vi "Leader.vi"   [LabVIEW 2016]
uses:
  <vilib>/NXT/Block Support/NXT_TimerIndex.ctl
  <vilib>/NXT/Block Support/NXT_OutputPort.ctl
  <vilib>/NXT/Subs/MotorOutput.ctl
  <vilib>/NXT/Dual Mode Library/Sensors/Reset_Timer.vi
  <vilib>/NXT/Dual Mode Library/Sensors/Read_Timer.vi
  <vilib>/NXT/Dual Mode Library/Motors/ResetMotor.vi
  <vilib>/NXT/Dual Mode Library/Motors/Rotation.vi
  <vilib>/NXT/NXTIO Xnodes/NXTIONodeSubVIs/NXTMoveMotors.vi
  <vilib>/NXT/Dual Mode Library/Display/drawNumber_float.vi
  <vilib>/NXT/NXTIO Xnodes/NXTIONodeSubVIs/NXTStopMotors.vi
  <vilib>/NXT/Dual Mode Library/Display/drawText.vi
  <vilib>/NXT/Dual Mode Library/Display/drawNumber.vi
  <vilib>/NXT/Dual Mode Library/Display/drawText_Right.vi
  <vilib>/NXT/Subs/LVHSConnector.ctl
  <vilib>/NXT/NXTIO Xnodes/AddressXNode/NXTIOAddress.xnode
  <vilib>/NXT/NXTIO Xnodes/NXTIOXNode/NXTIO.xnode
  <vilib>/NXT/LegoClasses/BrickReference/BrickReference.lvclass
types:
  T1 = typedef "NXT_TimerIndex.ctl" = u8
  T2 = typedef "LVHSConnector.ctl" = refnum<class "BrickReference.lvclass">
  T3 = typedef "NXT_OutputPort.ctl" = u8
  T4 = typedef "MotorOutput.ctl" = u8
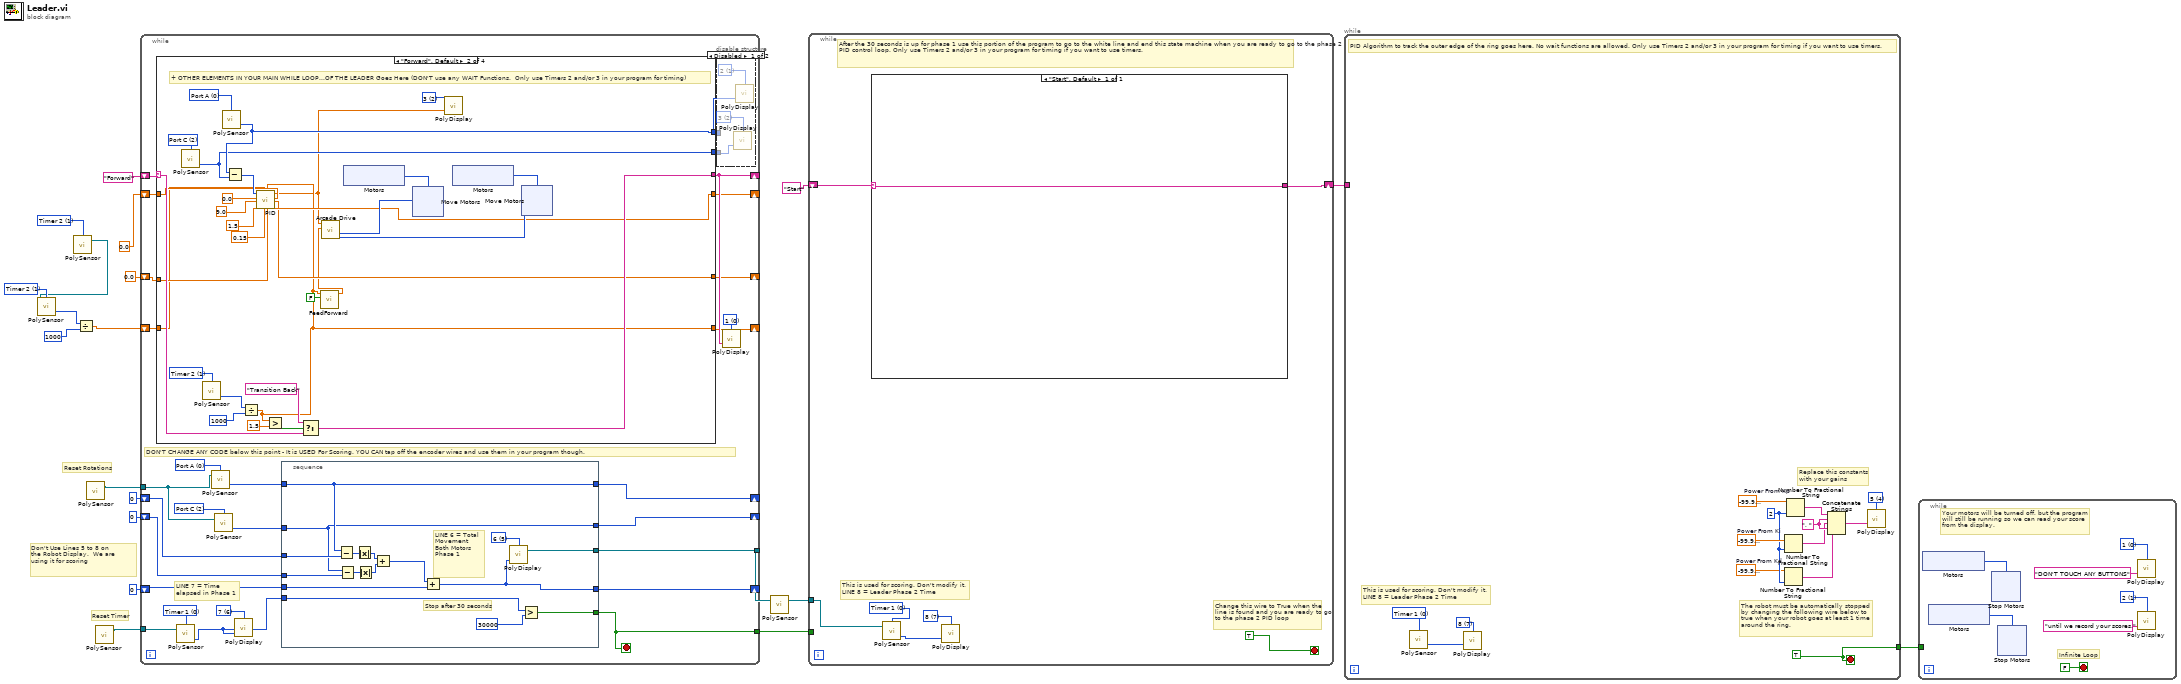
[diagram p0: block diagram]
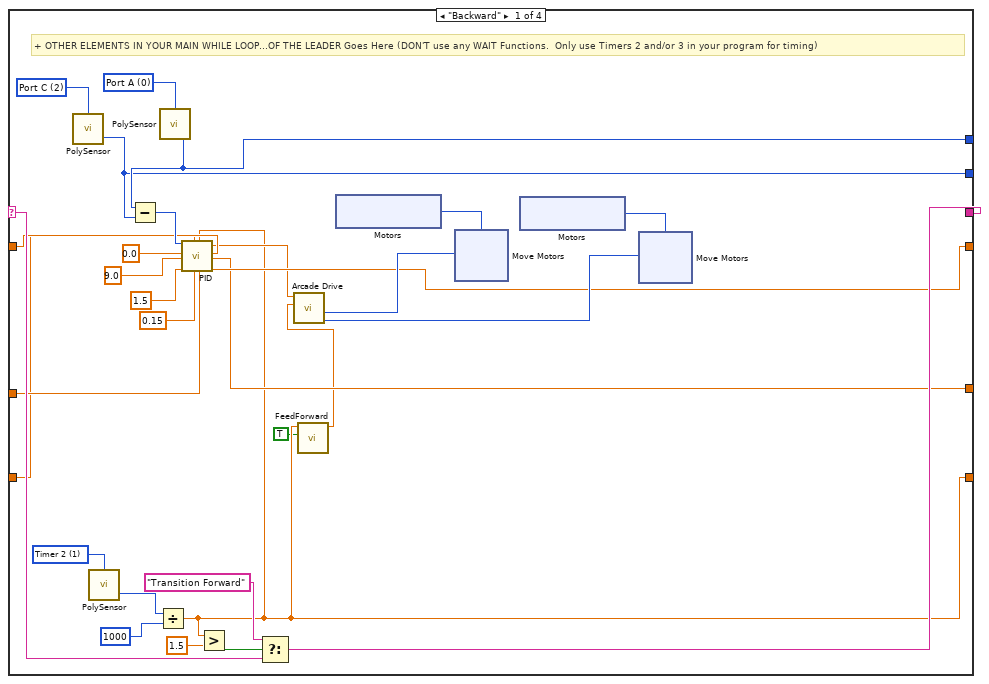
[diagram p3: hidden frame]
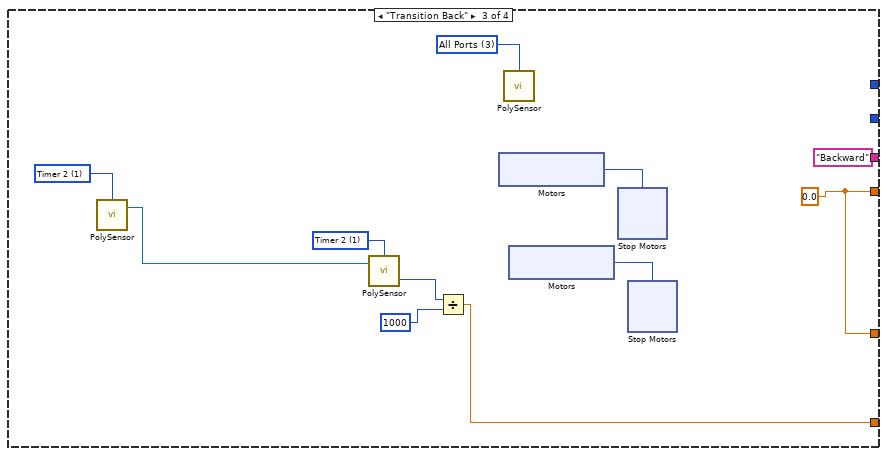
[diagram p4: hidden frame]
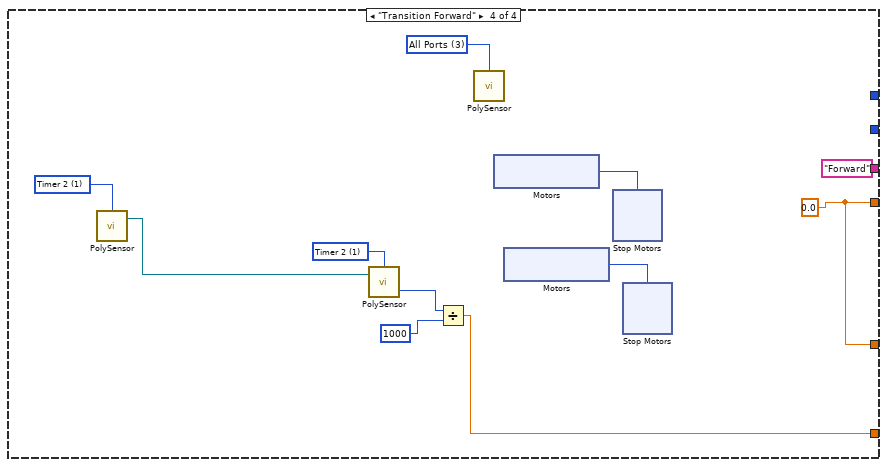
[diagram p5: hidden frame]
diagram:
  w4 = T1 1 items=["Timer 1", "Timer 2", "Timer 3"] ("Timer (Timer 1)")
  w8 = T1 1 items=["Timer 1", "Timer 2", "Timer 3"] ("Timer (Timer 1)")
  # "Don't Use Lines 5 to 8 on\nthe Robot Display.  We are \nusing it for scoring"
  # "Reset Timer"
  # "Reset Rotations"
  n1 = call-poly <vilib>:"PolySensor.vi"("Timer (Timer 1)"=w8) -> ("NXT/EV3"=w2:T2)  [unwired: 3 in]
  n2 = call-poly <vilib>:"PolySensor.vi"("NXT/EV3"=w2, "Timer (Timer 1)"=w4) -> ("Value (msec)"=w5:u32)  [unwired: 1 in, 1 out]
  n3 = Divide(x=w5, y=u32 1000) -> (x/y=w1:dbl)
  n4 = call-poly <vilib>:"PolySensor.vi"() -> ("NXT/EV3"=w16:T2)  [unwired: 4 in]
  n5 = call-poly <vilib>:"PolySensor.vi"() -> ("NXT/EV3"=w15:T2)  [unwired: 4 in]
  n6 = while {
    tunnel: w16 -> [w48]
    shift-right: [w40] -> _
    shift-left: 0 ("Angle of Rotation") -> [w42]
    shift-right: [w39] -> _
    shift-left: 0 ("Angle of Rotation") -> [w41]
    shift-right: [w46] -> _
    shift-left: 0 -> [w47]
    tunnel: w15 -> [w36]
    tunnel: [w45] -> w13
    shift-right: [w29] -> _
    shift-left: "Forward" -> [w38]
    tunnel: [w31] -> w12
    shift-right: [w27] -> _
    shift-left: 0.0 ("Accumulate In") -> [w28]
    shift-right: [w25] -> _
    shift-left: 0.0 ("Accumulate In") -> [w26]
    shift-right: [w23] -> _
    shift-left: w1 -> [w24]
    stop <- w45 stop-if-true
    w30 = i16 0 items=["1", "2", "3", "4", "5", "6", "7", "8", "9", "10", "11", "12"] ("Line")
    w33 = i16 6 items=["1", "2", "3", "4", "5", "6", "7", "8", "9", "10", "11", "12"] ("Line")
    w34 = T3 0 items=["Port A", "Port B", "Port C", "Port D"] ("Port (Port A)")
    w35 = T3 2 items=["Port A", "Port B", "Port C", "Port D"] ("Port (Port A)")
    w37 = T1 0 items=["Timer 1", "Timer 2", "Timer 3"] ("Timer (Timer 1)")
    # "DON'T CHANGE ANY CODE below this point - It is USED For Scoring. YOU CAN tap off the encoder wires and use them in your program though."
    # "LINE 7 = Time elapsed in Phase 1"
    n7 = case shown="\"Forward\", Default" w38 {
      selector: w38 -> [w77 w124 _ _]
      tunnel: [w78 w125 "Backward" ("t") "Forward" ("t")] -> w29
      tunnel: w28 -> [w63 w110 _ _]
      tunnel: [w61 w108 w154 w177] -> w27
      tunnel: w26 -> [w60 w107 _ _]
      tunnel: [w62 w109 w154 w177] -> w25
      tunnel: w24 -> [w59 w106 _ _]
      tunnel: [w55 w103 w149 w172] -> w23
      tunnel: [w58 w105 _ _] -> w22
      tunnel: [w57 w104 _ _] -> w21
      frame "Backward" {
        w72 = T3 2 items=["Port A", "Port B", "Port C", "Port D"] ("Port (Port A)")
        w73 = T3 0 items=["Port A", "Port B", "Port C", "Port D"] ("Port (Port A)")
        w80 = T1 1 items=["Timer 1", "Timer 2", "Timer 3"] ("Timer (Timer 1)")
        # "+ OTHER ELEMENTS IN YOUR MAIN WHILE LOOP...OF THE LEADER Goes Here (DON'T use any WAIT Functions.  Only use Timers 2 and/or 3 in your program for timing)"
        n8 = call-poly <vilib>:"PolySensor.vi"("Port (Port A)"=w72) -> ("Angle of Rotation"=w57:i32)  [unwired: 2 in, 1 out]
        n9 = call-poly <vilib>:"PolySensor.vi"("Timer (Timer 1)"=w80) -> ("Value (msec)"=w71:u32)  [unwired: 2 in, 1 out]
        n10 = Divide(x=w71, y=u32 1000) -> (x/y=w55:dbl)
        n11 = call-poly <vilib>:"PolySensor.vi"("Port (Port A)"=w73) -> ("Angle of Rotation"=w58:i32)  [unwired: 2 in, 1 out]
        n12 = Subtract(x=w58, y=w57) -> (x-y=w68:i32)
        n13 = call "PID.vi"("Sensor Input"=w68, "Setpoint"=0.0, "Kp"=9.0, "Ki"=1.5, "Prev Time"=w59, "Kd"=0.15, "Curr Time"=w55, "Accumulate In"=w63, "Previous Error"=w60) -> ("Output Val"=w56:dbl, "Accumulate Out"=w61:dbl, "Current Error"=w62:dbl)  [unwired: 5 in, 3 out]
        n14 = Greater?(x=w55, y=1.5) -> (0:w79:bool)
        n15 = Select(t="Transition Forward", s=w79, f=w77) -> (s? t:f=w78:string)
        n16 = call "FeedForward.vi"("backward?"=TRUE, "Current Time"=w55) -> ("f(t)"=w54:sgl)  [unwired: 9 in]
        n17 = call "Arcade Drive.vi"("Drive"=w54, "Rotate"=w56) -> ("Left Motor"=w74:i8, "Right Motor"=w75:i8)  [unwired: 8 in]
        n18 = xnode "Motors"() -> ("Motor"=w81:T3)
        n19 = xnode "Move Motors"("Power/Speed 1"=w75, "Motors"=w81) -> ()  [unwired: 1 in, 1 out]
        n20 = xnode "Motors"() -> ("Motor"=w82:T3)
        n21 = xnode "Move Motors"("Power/Speed 1"=w74, "Motors"=w82) -> ()  [unwired: 1 in, 1 out]
      }
      frame "Forward", Default {
        w99 = i16 2 items=["1", "2", "3", "4", "5", "6", "7", "8", "9", "10", "11", "12"] ("Line")
        w119 = T3 2 items=["Port A", "Port B", "Port C", "Port D"] ("Port (Port A)")
        w120 = T3 0 items=["Port A", "Port B", "Port C", "Port D"] ("Port (Port A)")
        w127 = T1 1 items=["Timer 1", "Timer 2", "Timer 3"] ("Timer (Timer 1)")
        # "+ OTHER ELEMENTS IN YOUR MAIN WHILE LOOP...OF THE LEADER Goes Here (DON'T use any WAIT Functions.  Only use Timers 2 and/or 3 in your program for timing)"
        n22 = call-poly <vilib>:"PolySensor.vi"("Port (Port A)"=w119) -> ("Angle of Rotation"=w104:i32)  [unwired: 2 in, 1 out]
        n23 = call-poly <vilib>:"PolySensor.vi"("Timer (Timer 1)"=w127) -> ("Value (msec)"=w118:u32)  [unwired: 2 in, 1 out]
        n24 = call-poly <vilib>:"PolySensor.vi"("Port (Port A)"=w120) -> ("Angle of Rotation"=w105:i32)  [unwired: 2 in, 1 out]
        n25 = Subtract(x=w105, y=w104) -> (x-y=w115:i32)
        n26 = Divide(x=w118, y=u32 1000) -> (x/y=w103:dbl)
        n27 = call "PID.vi"("Sensor Input"=w115, "Setpoint"=0.0, "Kp"=9.0, "Ki"=1.5, "Prev Time"=w106, "Kd"=0.15, "Curr Time"=w103, "Accumulate In"=w110, "Previous Error"=w107) -> ("Output Val"=w100:dbl, "Accumulate Out"=w108:dbl, "Current Error"=w109:dbl)  [unwired: 5 in, 3 out]
        n28 = Greater?(x=w103, y=1.5) -> (0:w126:bool)
        n29 = Select(t="Transition Back", s=w126, f=w124) -> (s? t:f=w125:string)
        n30 = call "FeedForward.vi"("backward?"=FALSE, "Current Time"=w103) -> ("f(t)"=w101:sgl)  [unwired: 9 in]
        n31 = call "Arcade Drive.vi"("Drive"=w101, "Rotate"=w100) -> ("Left Motor"=w121:i8, "Right Motor"=w122:i8)  [unwired: 8 in]
        n32 = xnode "Motors"() -> ("Motor"=w128:T3)
        n33 = xnode "Move Motors"("Power/Speed 1"=w122, "Motors"=w128) -> ()  [unwired: 1 in, 1 out]
        n34 = call-poly <vilib>:"PolyDisplay.vi"("number"=w100, "Line"=w99) -> ()  [unwired: 2 in, 1 out]
        n35 = xnode "Motors"() -> ("Motor"=w129:T3)
        n36 = xnode "Move Motors"("Power/Speed 1"=w121, "Motors"=w129) -> ()  [unwired: 1 in, 1 out]
      }
      frame "Transition Back" {
        w148 = T4 3 items=["Port A"=0, "Port B"=1, "Port C"=2, "Ports A & B"=4, "Ports A & C"=5, "Ports B & C"=6, "All Ports"=3] ("Port (All Ports)")
        w152 = T1 1 items=["Timer 1", "Timer 2", "Timer 3"] ("Timer (Timer 1)")
        w154 = 0.0 ("Accumulate In")
        w156 = T1 1 items=["Timer 1", "Timer 2", "Timer 3"] ("Timer (Timer 1)")
        n37 = call-poly <vilib>:"PolySensor.vi"("Timer (Timer 1)"=w156) -> ("NXT/EV3"=w150:T2)  [unwired: 3 in]
        n38 = call-poly <vilib>:"PolySensor.vi"("NXT/EV3"=w150, "Timer (Timer 1)"=w152) -> ("Value (msec)"=w151:u32)  [unwired: 1 in, 1 out]
        n39 = Divide(x=w151, y=u32 1000) -> (x/y=w149:dbl)
        n40 = xnode "Motors"() -> ("Motor"=w147:T3)
        n41 = call-poly <vilib>:"PolySensor.vi"("Port (All Ports)"=w148) -> ()  [unwired: 3 in, 1 out]
        n42 = xnode "Motors"() -> ("Motor"=w146:T3)
        n43 = xnode "Stop Motors"("Motors"=w147) -> ()  [unwired: 1 in, 1 out]
        n44 = xnode "Stop Motors"("Motors"=w146) -> ()  [unwired: 1 in, 1 out]
      }
      frame "Transition Forward" {
        w171 = T4 3 items=["Port A"=0, "Port B"=1, "Port C"=2, "Ports A & B"=4, "Ports A & C"=5, "Ports B & C"=6, "All Ports"=3] ("Port (All Ports)")
        w175 = T1 1 items=["Timer 1", "Timer 2", "Timer 3"] ("Timer (Timer 1)")
        w177 = 0.0 ("Accumulate In")
        w179 = T1 1 items=["Timer 1", "Timer 2", "Timer 3"] ("Timer (Timer 1)")
        n45 = call-poly <vilib>:"PolySensor.vi"("Timer (Timer 1)"=w179) -> ("NXT/EV3"=w173:T2)  [unwired: 3 in]
        n46 = call-poly <vilib>:"PolySensor.vi"("NXT/EV3"=w173, "Timer (Timer 1)"=w175) -> ("Value (msec)"=w174:u32)  [unwired: 1 in, 1 out]
        n47 = Divide(x=w174, y=u32 1000) -> (x/y=w172:dbl)
        n48 = call-poly <vilib>:"PolySensor.vi"("Port (All Ports)"=w171) -> ()  [unwired: 3 in, 1 out]
        n49 = xnode "Motors"() -> ("Motor"=w170:T3)
        n50 = xnode "Motors"() -> ("Motor"=w169:T3)
        n51 = xnode "Stop Motors"("Motors"=w170) -> ()  [unwired: 1 in, 1 out]
        n52 = xnode "Stop Motors"("Motors"=w169) -> ()  [unwired: 1 in, 1 out]
      }
    }
    n53 = call-poly <vilib>:"PolySensor.vi"("NXT/EV3"=w36, "Timer (Timer 1)"=w37) -> ("Value (msec)"=w32:u32)  [unwired: 1 in, 1 out]
    n54 = call-poly <vilib>:"PolySensor.vi"("NXT/EV3"=w48, "Port (Port A)"=w34) -> ("Angle of Rotation"=w44:i32)  [unwired: 1 in, 1 out]
    n55 = call-poly <vilib>:"PolySensor.vi"("NXT/EV3"=w48, "Port (Port A)"=w35) -> ("Angle of Rotation"=w43:i32)  [unwired: 1 in, 1 out]
    n56 = call-poly <vilib>:"PolyDisplay.vi"("number"=w32, "Line"=w33) -> ()  [unwired: 2 in, 1 out]
    n57 = stacked-sequence {
      tunnel: w47 -> [w207]
      tunnel: [w194] -> w46
      tunnel: w32 -> [w205]
      tunnel: [w204] -> w45
      tunnel: w44 -> [w197]
      tunnel: w43 -> [w196]
      tunnel: w42 -> [w199]
      tunnel: w41 -> [w198]
      tunnel: [w197] -> w40
      tunnel: [w196] -> w39
      tunnel: [w192] -> w31
      frame #0 {
        w193 = i16 5 items=["1", "2", "3", "4", "5", "6", "7", "8", "9", "10", "11", "12"] ("Line")
        # "LINE 6 = Total\nMovement\nBoth Motors\nPhase 1"
        # "Stop after 30 seconds"
        n58 = Subtract(x=w197, y=w199) -> (x-y=w203:i32)
        n59 = Subtract(x=w196, y=w198) -> (x-y=w202:i32)
        n60 = Absolute Value(x=w203) -> (abs(x)=w201:i32)
        n61 = Absolute Value(x=w202) -> (abs(x)=w200:i32)
        n62 = Add(x=w201, y=w200) -> (x+y=w195:i32)
        n63 = Add(x=w195, y=w207) -> (x+y=w194:i32)
        n64 = call-poly <vilib>:"PolyDisplay.vi"("number"=w194, "Line"=w193) -> ("NXT/EV3"=w192:T2)  [unwired: 2 in]
        n65 = Greater?(x=w205, y=u32 30000 ("Value (msec)")) -> (0:w204:bool)
      }
    }
    n66 = disable-structure shown="Disabled" {
      disable-tunnel: w22 -> [w51 _]
      disable-tunnel: w21 -> [w49 _]
      frame Disabled {
        w50 = i16 2 items=["1", "2", "3", "4", "5", "6", "7", "8", "9", "10", "11", "12"] ("Line")
        w52 = i16 1 items=["1", "2", "3", "4", "5", "6", "7", "8", "9", "10", "11", "12"] ("Line")
        n67 = call-poly <vilib>:"PolyDisplay.vi"("number"=w49, "Line"=w50) -> ()  [unwired: 2 in, 1 out]
        n68 = call-poly <vilib>:"PolyDisplay.vi"("number"=w51, "Line"=w52) -> ()  [unwired: 2 in, 1 out]
      }
      frame Enabled {
      }
    }
    n69 = call-poly <vilib>:"PolyDisplay.vi"("Text"=w29, "Line"=w30) -> ()  [unwired: 2 in, 1 out]
  }
  n70 = call-poly <vilib>:"PolySensor.vi"("NXT/EV3"=w12) -> ("NXT/EV3"=w11:T2)  [unwired: 3 in]
  n71 = while {
    shift-right: [w213] -> w10
    shift-left: "Start" -> [w214]
    tunnel: w13 -> [_]
    tunnel: w11 -> [w209]
    stop <- TRUE stop-if-true
    w211 = i16 7 items=["1", "2", "3", "4", "5", "6", "7", "8", "9", "10", "11", "12"] ("Line")
    w212 = T1 0 items=["Timer 1", "Timer 2", "Timer 3"] ("Timer (Timer 1)")
    # "This is used for scoring. Don't modify it.\nLINE 8 = Leader Phase 2 Time"
    # "Change this wire to True when the line is found and you are ready to go to the phase 2 PID loop"
    # "After the 30 seconds is up for phase 1 use this portion of the program to go to the white line and end this state machine when you are ready to go to the phase 2 PID control loop. Only use Timers 2 and/or 3 in your program for timing if you want to use timers."
    n72 = case shown="\"Start\", Default" w214 {
      selector: w214 -> [w215]
      tunnel: [w215] -> w213
      frame "Start", Default {
      }
    }
    n73 = call-poly <vilib>:"PolySensor.vi"("NXT/EV3"=w209, "Timer (Timer 1)"=w212) -> ("Value (msec)"=w210:u32)  [unwired: 1 in, 1 out]
    n74 = call-poly <vilib>:"PolyDisplay.vi"("number"=w210, "Line"=w211) -> ()  [unwired: 2 in, 1 out]
  }
  n75 = while {
    tunnel: [w226] -> w9
    tunnel: w10 -> [_]
    stop <- w226 stop-if-true
    w219 = ", " ("string")
    w222 = i16 2 ("precision (6)")
    w221 = sgl -99.9  # Power From Kd
    w223 = sgl -99.9  # Power From Ki
    w224 = sgl -99.9  # Power From Kp
    w225 = i16 4 items=["1", "2", "3", "4", "5", "6", "7", "8", "9", "10", "11", "12"] ("Line")
    w226 = TRUE
    w227 = i16 7 items=["1", "2", "3", "4", "5", "6", "7", "8", "9", "10", "11", "12"] ("Line")
    w229 = T1 0 items=["Timer 1", "Timer 2", "Timer 3"] ("Timer (Timer 1)")
    # "Replace this constants\nwith your gains"
    # "This is used for scoring. Don't modify it.\nLINE 8 = Leader Phase 2 Time"
    # "The robot must be automatically stopped\nby changing the following wire below to\ntrue when your robot goes at least 1 time\naround the ring."
    # "PID Algorithm to track the outer edge of the ring goes here. No wait functions are allowed. Only use Timers 2 and/or 3 in your program for timing if you want to use timers."
    n76 = call-poly <vilib>:"PolySensor.vi"("Timer (Timer 1)"=w229) -> ("Value (msec)"=w228:u32)  [unwired: 2 in, 1 out]
    n77 = call-poly <vilib>:"PolyDisplay.vi"("number"=w228, "Line"=w227) -> ()  [unwired: 2 in, 1 out]
    n78 = Number To Fractional String(number=w223, precision (6)=w222) -> (F-format string=w218:string)  [unwired: 2 in]
    n79 = Number To Fractional String(number=w221, precision (6)=w222) -> (F-format string=w217:string)  [unwired: 2 in]
    n80 = Number To Fractional String(number=w224, precision (6)=w222) -> (F-format string=w220:string)  [unwired: 2 in]
    n81 = Concatenate Strings(w220, w219, w218, w219, w217) -> (w216:string)
    n82 = call-poly <vilib>:"PolyDisplay.vi"("Text"=w216, "Line"=w225) -> ()  [unwired: 2 in, 1 out]
  }
  n83 = while {
    tunnel: w9 -> [_]
    stop <- FALSE stop-if-true
    w233 = i16 1 items=["1", "2", "3", "4", "5", "6", "7", "8", "9", "10", "11", "12"] ("Line")
    w232 = i16 0 items=["1", "2", "3", "4", "5", "6", "7", "8", "9", "10", "11", "12"] ("Line")
    # "Your motors will be turned off, but the program\nwill still be running so we can read your score\nfrom the display."
    # "Infinite Loop"
    n84 = xnode "Motors"() -> ("Motor"=w235:T3)
    n85 = xnode "Motors"() -> ("Motor"=w234:T3)
    n86 = xnode "Stop Motors"("Motors"=w235) -> ()  [unwired: 1 in, 1 out]
    n87 = xnode "Stop Motors"("Motors"=w234) -> ()  [unwired: 1 in, 1 out]
    n88 = call-poly <vilib>:"PolyDisplay.vi"("Text"="DON'T TOUCH ANY BUTTONS", "Line"=w232) -> ()  [unwired: 2 in, 1 out]
    n89 = call-poly <vilib>:"PolyDisplay.vi"("Text"="until we record your scores.", "Line"=w233) -> ()  [unwired: 2 in, 1 out]
  }
